vi "Read Table Configuration.vi"(8 "error in (no error)":errorcluster, 11 "Basic Table in":refnum<class "Basic Table.lvclass">) -> (0 "error out":errorcluster, 2 "Table Configuration":refnum<class "Table Configuration Interface.lvclass">, 3 "Basic Table out":refnum<class "Basic Table.lvclass">)   [LabVIEW 2020, in "Table.lvlib" / "Basic Table.lvclass"]
uses:
  Basic Table.lvclass
  Table Configuration Interface/Table Configuration Interface.lvclass
  Basic Table.lvclass/Basic Table.ctl
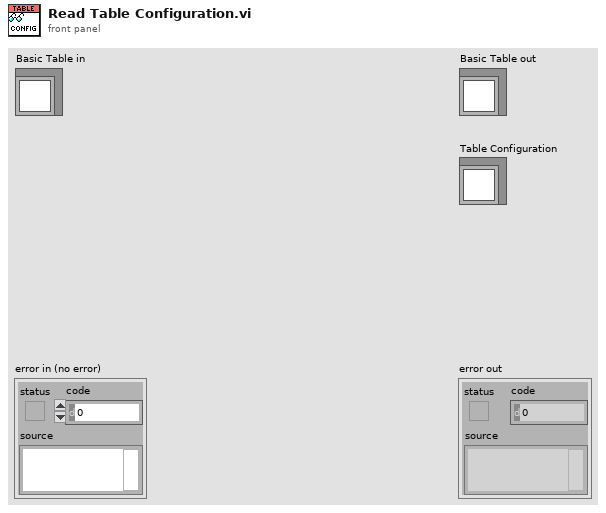
[diagram p1: front panel]
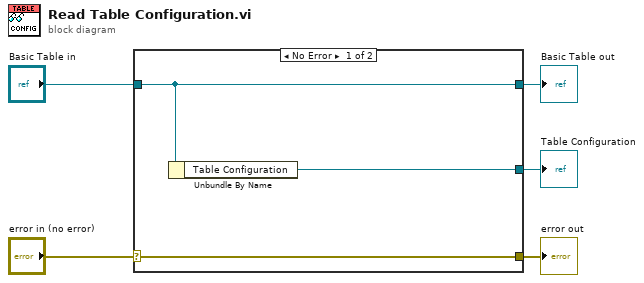
[diagram p0: block diagram]
diagram:
  n1 = case shown="No Error" "error in (no error)" {
    selector: "error in (no error)" -> [w8 w9]
    tunnel: [w8 w9] -> w4
    tunnel: [w7 w10] -> w2
    tunnel: "Basic Table in" -> [w7 w10]
    tunnel: [w6 _] -> w1
    frame No Error {
      n2 = Unbundle By Name(w7) -> ("Table Configuration"=w6:refnum<class "Table Configuration Interface.lvclass">)
    }
    frame Error {
    }
  }
  "error out" <- w4
  "Basic Table out" <- w2
  "Table Configuration" <- w1
